vi "measure.vi"(6 "Nmsr":i16, 8 "error in (no error)":errorcluster, 9 "Wnd":i32, 10 "Device":i32, 11 "SEDSpectrometer in":refnum<class "FiberSpectrograph.lvclass">) -> (0 "error out":errorcluster, 2 "Output Value":i32, 3 "SEDSpectrometer out":refnum<class "FiberSpectrograph.lvclass">)   [LabVIEW 2016, in "FiberSpectrograph.lvclass"]
uses:
  FiberSpectrograph.lvclass
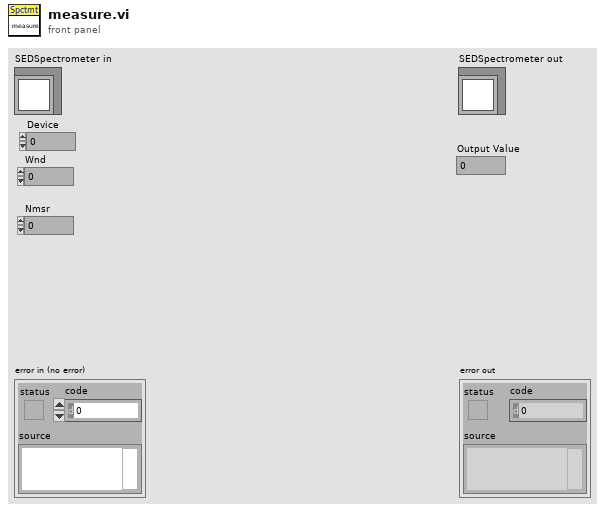
[diagram p1: front panel]
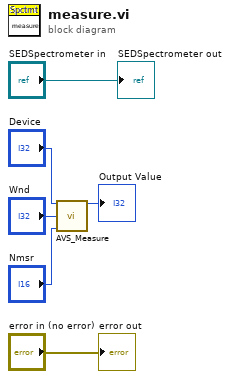
[diagram p0: block diagram]
diagram:
  n1 = call "AVS_Measure.vi"("a_hDevice"="Device", "a_hWnd"="Wnd", "a_Nmsr"="Nmsr") -> ("Output Value"=→"Output Value":i32)  [unwired: 12 in]
  "error out" <- "error in (no error)"
  "SEDSpectrometer out" <- "SEDSpectrometer in"
